vi "Cache.Max Block Count.vi"(8 "error in (no error)":errorcluster, 11 "Cache in":refnum<class "Cache.lvclass">) -> (0 "error out":errorcluster, 2 "largest block count":u64, 3 "Cache out":refnum<class "Cache.lvclass">)   [LabVIEW 2017, in "DSF Core.lvlib" / "Cache.lvclass"]
uses:
  Cache.lvclass
  Cache.lvclass/Cache.ctl
  Transfer/Transfer Group.lvclass
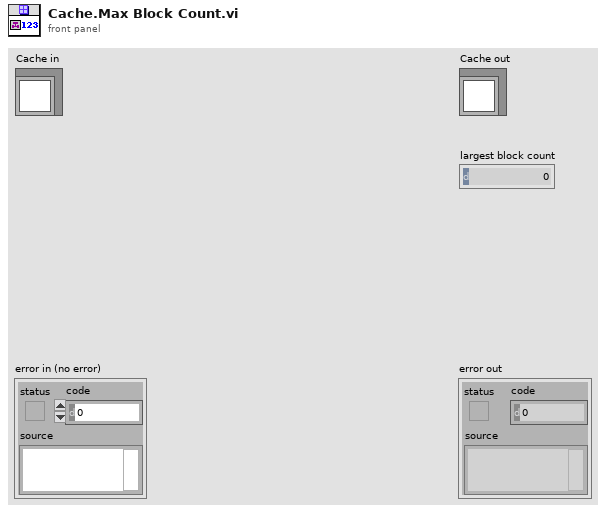
[diagram p1: front panel]
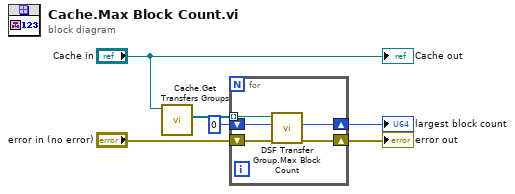
[diagram p0: block diagram]
diagram:
  n1 = call "Cache.Get Transfers Groups.vi"("Cache in"="Cache in") -> ("Transfers Groups"=w5:refnum<class "Transfer Group.lvclass">[])  [unwired: 9 in, 1 out]
  n2 = for {
    tunnel: w5 -> [w11] mode=indexing
    shift-right: [w7] -> w3
    shift-left: u64 0 ("max channel count") -> [w10]
    shift-right: [w8] -> w1
    shift-left: "error in (no error)" -> [w9]
    n3 = call "DSF Transfer Group.Max Block Count.vi"("error in (no error)"=w9, "previous block count (0)"=w10, "Transfer Group in"=w11) -> ("error out"=w8:errorcluster, "largest block count"=w7:u64)  [unwired: 6 in, 1 out]
  }
  "error out" <- w1
  "largest block count" <- w3
  "Cache out" <- "Cache in"
